vi "RPC Method TemperatureControllerService_Measure.vi"(8 "error in (no error)":errorcluster, 11 "OOP Server in":refnum<class "TempController_server.lvclass">) -> (0 "error out":errorcluster, 3 "OOP Server out":refnum<class "TempController_server.lvclass">)   [LabVIEW 2019, in "TempController_server.lvlib" / "TempController_server.lvclass"]
uses:
  TempController_server.lvclass
  TempController_server.lvclass/TempController_server.ctl
  Temperature Controller/Temperature Controller.lvclass
  RPC Messages/MeasureResponse/MeasureResponse_Data.ctl
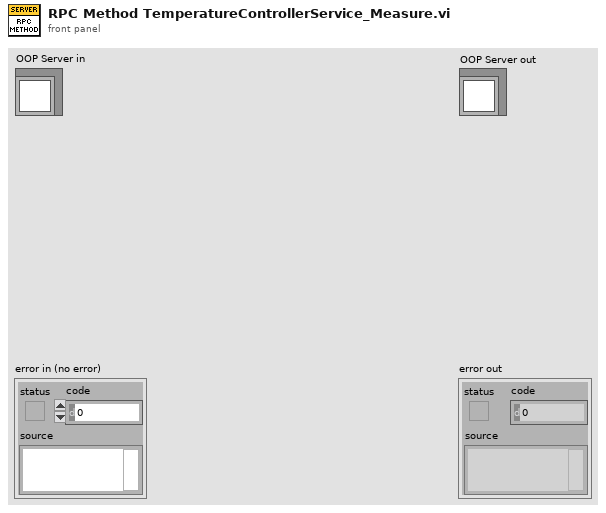
[diagram p1: front panel]
types:
  T1 = typedef "TempController_server.lvlib/TempController_server.lvclass/MeasureResponse_Data.ctl" = cluster{"temperature":dbl}
  T2 = typedef "TempController_server.lvlib/TempController_server.lvclass/Server Internal UEs.ctl" = cluster{"TemperatureControllerService_Measure Internal UE":refnum<user-event>, "TemperatureControllerService_Configure Internal UE":refnum<user-event>}
  T3 = typedef "TempController_server.lvlib/TempController_server.lvclass/Server gRPC UEs.ctl" = cluster{"TemperatureControllerService_Measure gRPC UE":refnum<user-event>, "TemperatureControllerService_Configure gRPC UE":refnum<user-event>}
  T4 = typedef "gprc-lvsupport-release.lvlib/grpcId.ctl" = u64
  T5 = typedef "TempController_server.lvlib/TempController_server.lvclass/MeasureRequest_Data.ctl" = cluster{"unit":i32}
  T6 = typedef "TempController_server.lvlib/TempController_server.lvclass/Server State Data.ctl" = cluster{"controller":refnum<class "Temperature Controller.lvclass">}
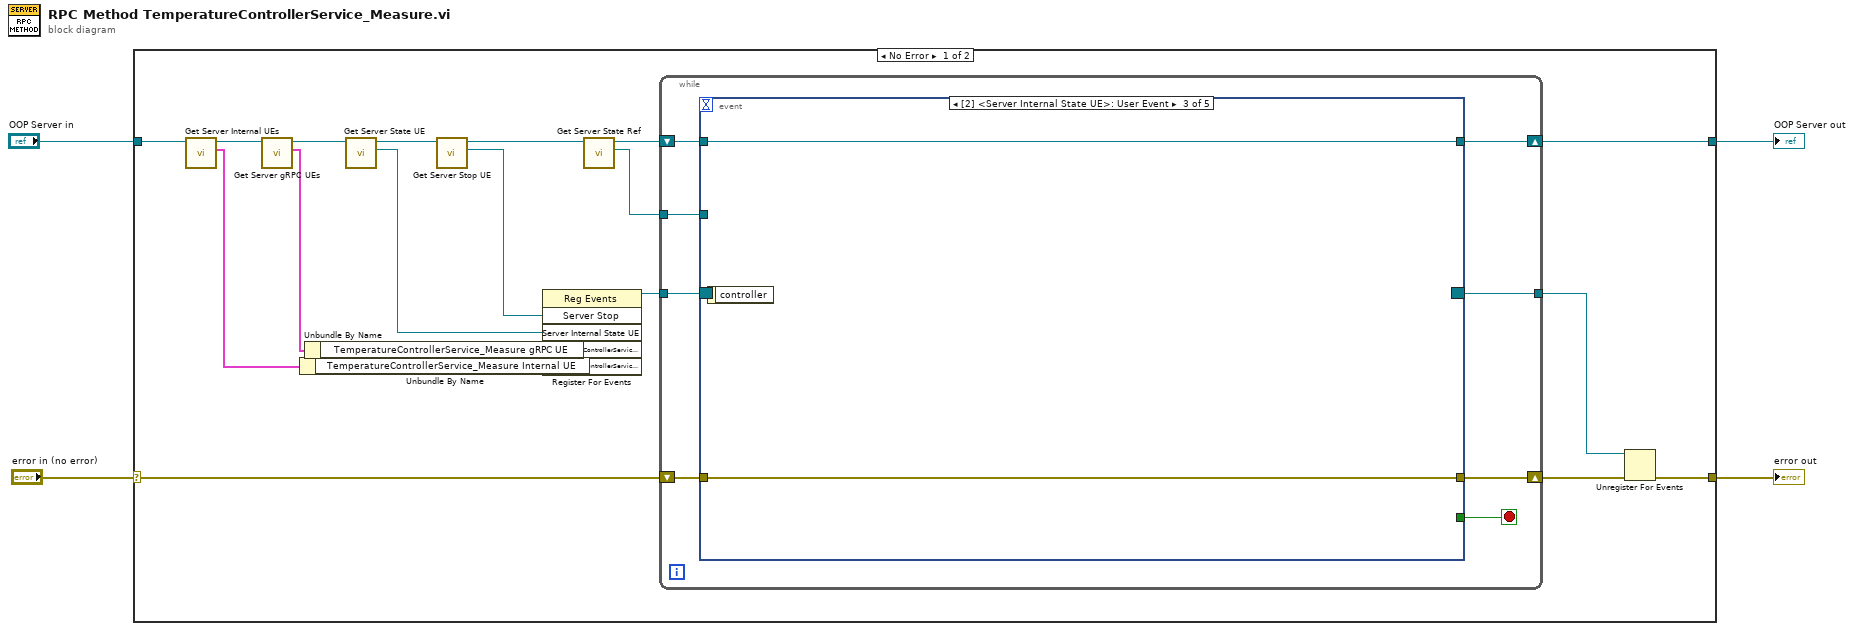
[diagram p0: block diagram]
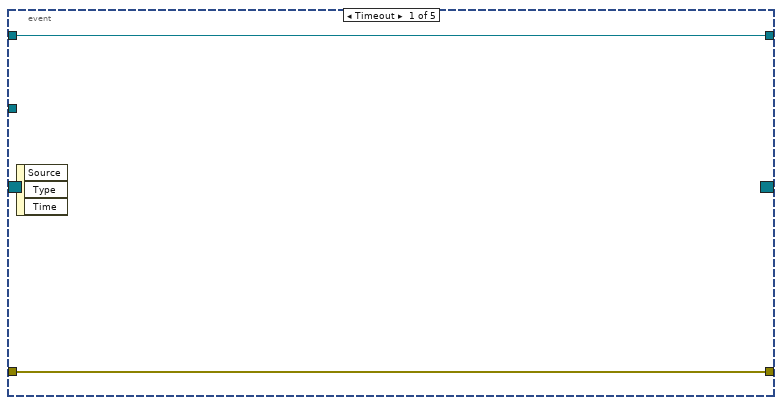
[diagram p2: hidden frame]
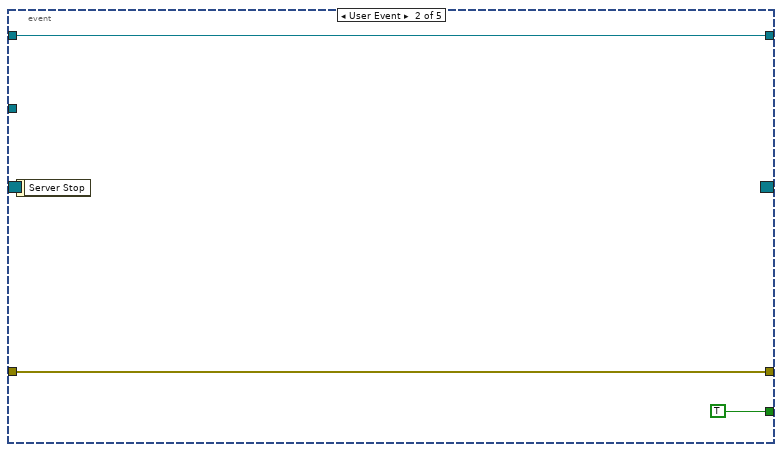
[diagram p3: hidden frame]
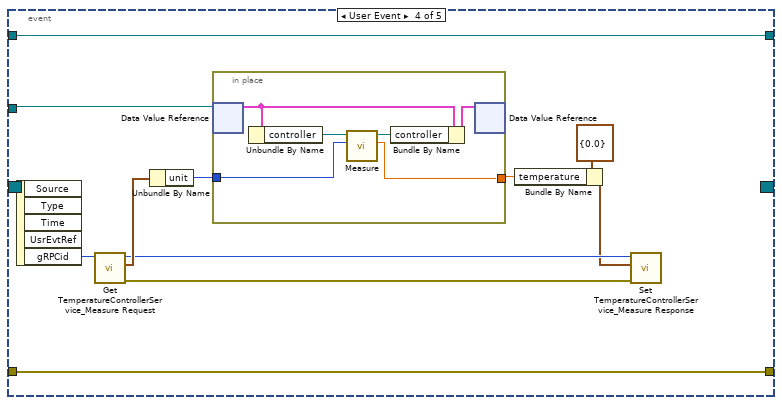
[diagram p4: hidden frame]
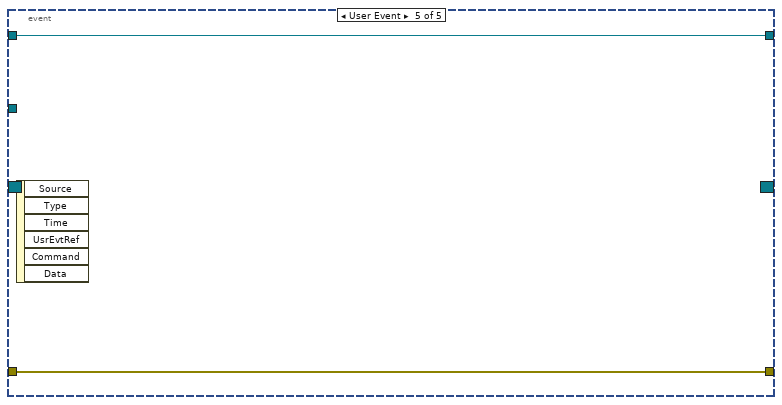
[diagram p5: hidden frame]
diagram:
  n1 = case shown="No Error" "error in (no error)" {
    selector: "error in (no error)" -> [w19 w59]
    tunnel: [w17 w59] -> w3
    tunnel: "OOP Server in" -> [w21 w58]
    tunnel: [w8 w58] -> w1
    frame No Error {
      n2 = call "Get Server Internal UEs.vi"("OOP Server in"=w21) -> ("Server Internal UEs"=w13:T2, "OOP Server out"=w20:refnum<class "TempController_server.lvclass">)  [unwired: 9 in]
      n3 = call "Get Server gRPC UEs.vi"("OOP Server in"=w20) -> ("Server RPC Methods"=w15:T3, "OOP Server out"=w11:refnum<class "TempController_server.lvclass">)  [unwired: 9 in]
      n4 = Unbundle By Name ("Unbundle Internal UE")(w13) -> ("TemperatureControllerService_Measure Internal UE"=w12:refnum<user-event>)
      n5 = Unbundle By Name ("Unbundle gRPC UE")(w15) -> ("TemperatureControllerService_Measure gRPC UE"=w14:refnum<user-event>)
      n6 = call "Get Server State UE.vi"("Template Server in"=w11) -> ("Server Internal State UE"=w9:refnum<user-event>, "Template Server out"=w10:refnum<class "TempController_server.lvclass">)  [unwired: 9 in]
      n7 = call "Get Server Stop UE.vi"("OOP Server in"=w10) -> ("Server Stop"=w23:refnum<user-event>, "OOP Server out"=w7:refnum<class "TempController_server.lvclass">)  [unwired: 9 in]
      n8 = register-events(w23, w9, w14, w12) -> (reference out=w22:refnum<event-registration>)  [unwired: 2 in, 1 out]
      n9 = call "Get Server State Ref.vi"("Template Server in"=w7) -> ("Server State Ref"=w5:refnum<data-value>, "Template Server out"=w6:refnum<class "TempController_server.lvclass">)  [unwired: 9 in]
      n10 = while {
        tunnel: w22 -> [w31]
        tunnel: [w27] -> w16
        shift-right: [w28] -> w18
        shift-left: w19 -> [w29]
        shift-right: [w25] -> w8
        shift-left: w6 -> [w26]
        tunnel: w5 -> [w24]
        stop <- w30 stop-if-true
        n11 = event "RPC Method Event Structure" shown="[2] <Server Internal State UE>: User Event" {
          selector: w31 -> [_ _ _ _ _]
          dyn-events: [_ _ _ _ _] -> w27
          timeout: _ -> [_ _ _ _ _]
          tunnel: [_ TRUE _ _ _] -> w30
          tunnel: w29 -> [w33 w35 w38 w49 w57]
          tunnel: [w33 w35 w38 w49 w57] -> w28
          tunnel: w26 -> [w32 w34 w37 w48 w56]
          tunnel: [w32 w34 w37 w48 w56] -> w25
          tunnel: w24 -> [_ _ _ w45 _]
          event Timeout {
            n12 = event-data() -> ()  [unwired: 1 in, 3 out]
          }
          event User Event {
            n13 = event-data() -> ()  [unwired: 1 in, 1 out]
          }
          event User Event {
            n14 = event-data() -> ()  [unwired: 1 in, 1 out]
          }
          event User Event {
            n15 = event-data() -> ("gRPCid"=w47:T4)  [unwired: 1 in, 4 out]
            n16 = call "Get TemperatureControllerService_Measure Request.vi"("gRPCid in"=w47) -> ("error out"=w39:errorcluster, "Message Data"=w46:T5, "gRPCid out"=w43:T4)  [unwired: 8 in]
            n17 = Unbundle By Name(w46) -> ("unit"=w44:i32)
            n18 = in-place {
              in-place-border: w44 -> [w53]
              in-place-border: [w50] -> w40
              n19 = in-place-dvr #1(w45) -> (w55:T6)  [unwired: 1 out]
              n20 = Unbundle By Name(w55) -> ("controller"=w54:refnum<class "Temperature Controller.lvclass">)
              n21 = call "Measure.vi"("unit"=w53, "controller in"=w54) -> ("measurement"=w50:dbl, "controller out"=w51:refnum<class "Temperature Controller.lvclass">)  [unwired: 7 in, 1 out]
              n22 = Bundle By Name(cluster=w55, "controller"=w51) -> (w52:T6)
              n23 = in-place-dvr #1(w52) -> ()  [unwired: 2 out]
            }
            n24 = Bundle By Name(cluster=T1 {"temperature"=0.0} ("Message Data"), "temperature"=w40) -> (w41:T1)
            n25 = call "Set TemperatureControllerService_Measure Response.vi"("error in (no error)"=w39, "Message Data"=w41, "gRPCid in"=w43) -> ()  [unwired: 8 in, 1 out]
          }
          event User Event {
            n26 = event-data() -> ()  [unwired: 1 in, 6 out]
          }
        }
      }
      n27 = Unregister For Events(event registration refnum=w16, error in=w18) -> (error out=w17:errorcluster)
    }
    frame Error {
    }
  }
  "error out" <- w3
  "OOP Server out" <- w1
